vi "Inst_K2002.vi"(8 "error in":errorcluster, 10 "All Message Queues in":T1, 11 "Prueba31 in":refnum<class "Prueba06.lvclass">) -> (0 "error out":errorcluster)   [LabVIEW 2019, in "Prueba06.lvclass"]
uses:
  Prueba06.lvclass
  QMH/Message Queue/All Message Queues.ctl
  QMH/Message Queue/Message Cluster.ctl
  Prueba06.lvclass/Prueba06.ctl
  <vilib>/Utility/error.llb/Error Cluster From Error Code.vi
  QMH/Message Queue/Enqueue Message (Single).vi
  <vilib>/ErrorRing/Error Ring.xnode
  QMH/Message Queue/Message Queue.lvlib
  Instrumento/Keithley2002/Keithley2002.lvclass
panel:
  out "All States":string[](array[string])
  out "Actual State":string
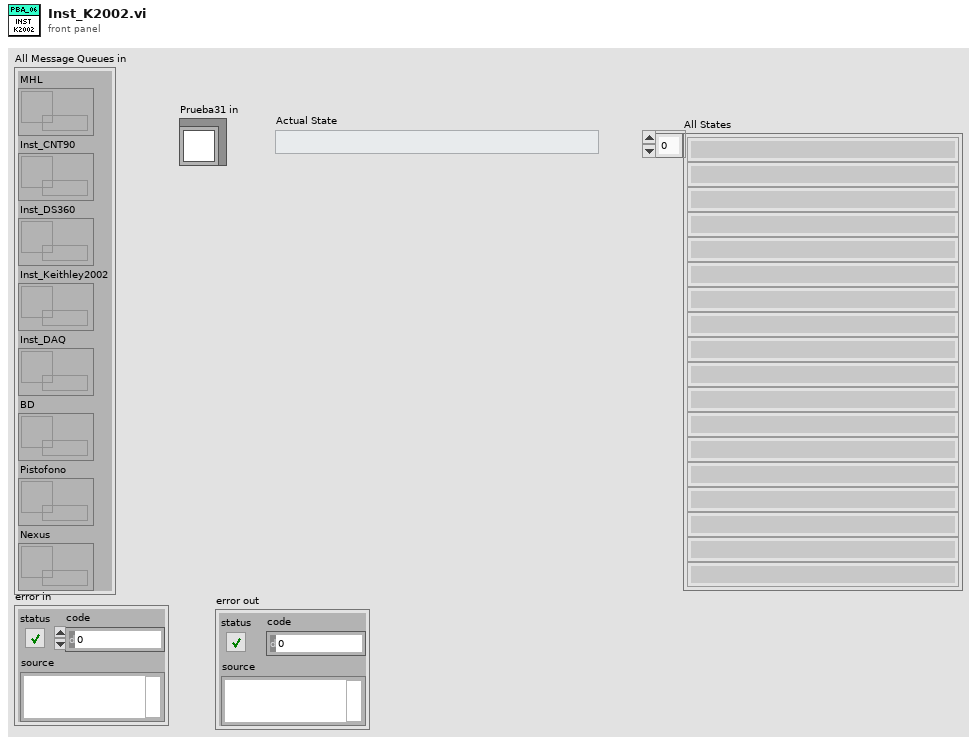
[diagram p1: front panel]
types:
  T1 = typedef "Message Queue.lvlib/All Message Queues.ctl" = cluster{"MHL":refnum<queue>, "Inst_CNT90":refnum<queue>, "Inst_DS360":refnum<queue>, "Inst_Keithley2002":refnum<queue>, "Inst_DAQ":refnum<queue>, "BD":refnum<queue>, "Pistofono":refnum<queue>, "Nexus":refnum<queue>}
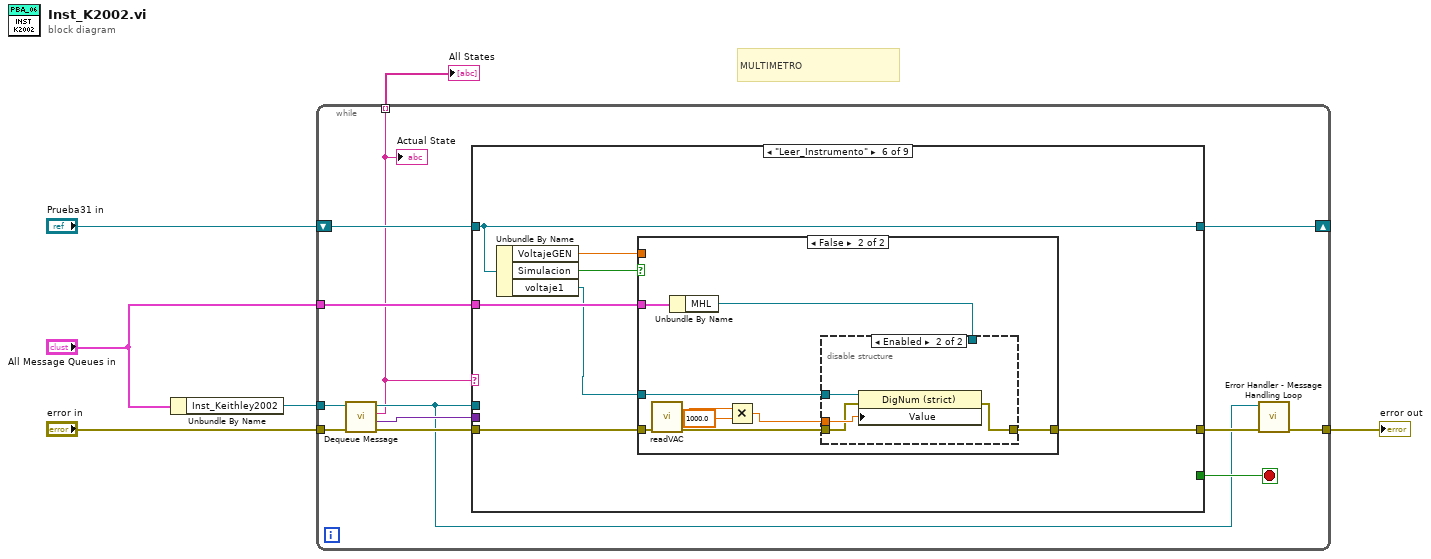
[diagram p0: block diagram]
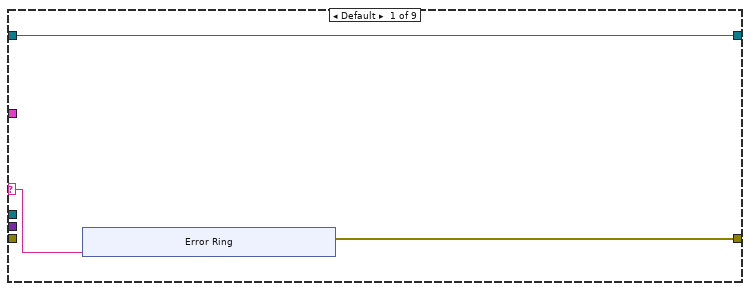
[diagram p2: hidden frame]
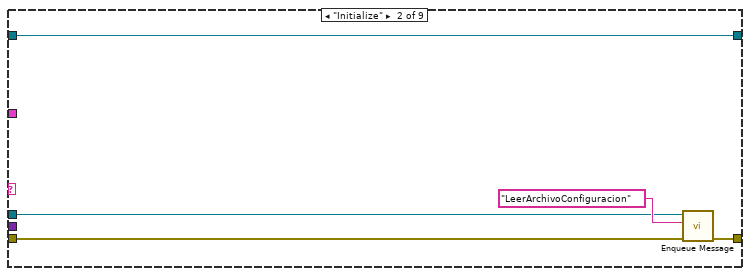
[diagram p3: hidden frame]
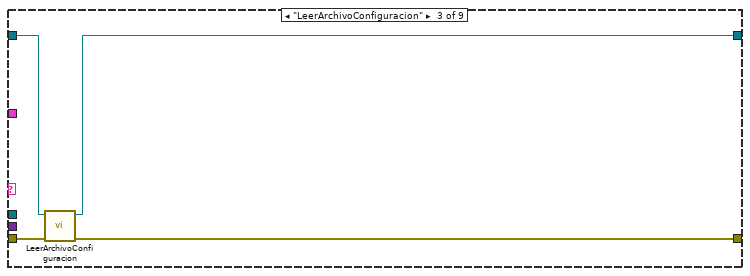
[diagram p4: hidden frame]
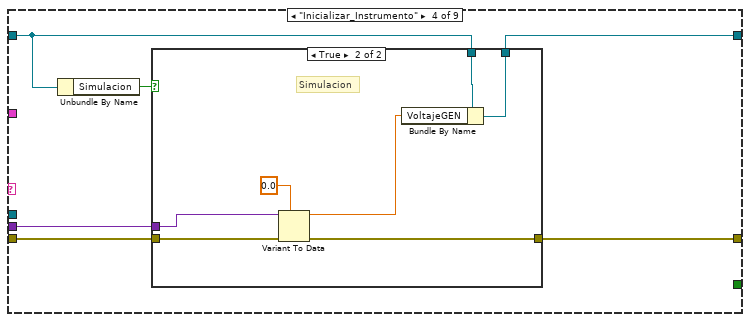
[diagram p5: hidden frame]
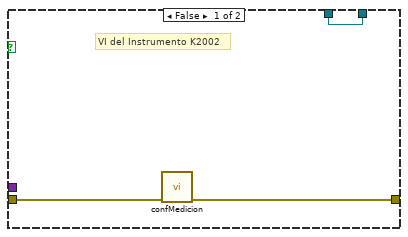
[diagram p6: hidden frame]
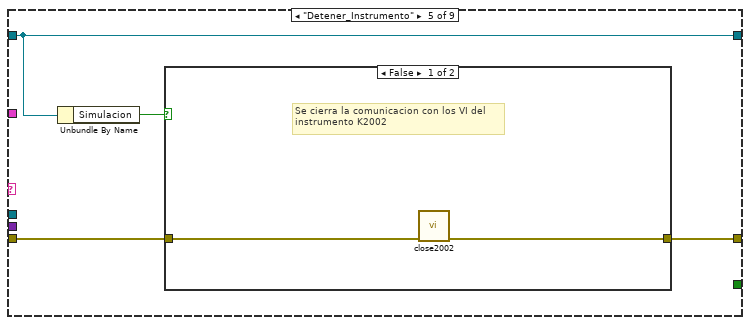
[diagram p7: hidden frame]
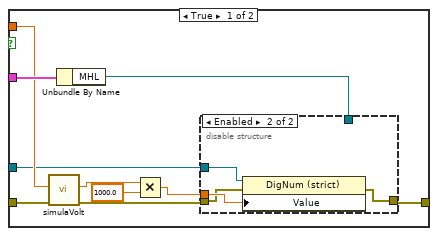
[diagram p9: hidden frame]
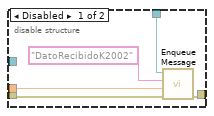
[diagram p10: hidden frame]
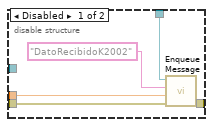
[diagram p11: hidden frame]
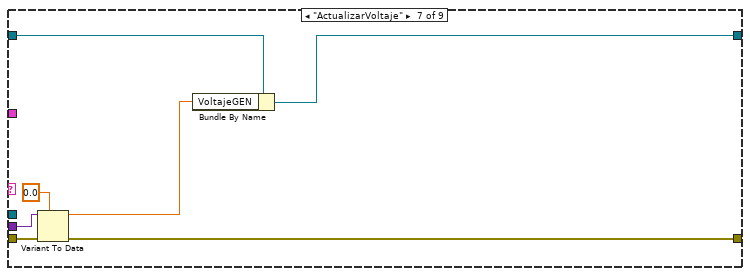
[diagram p12: hidden frame]
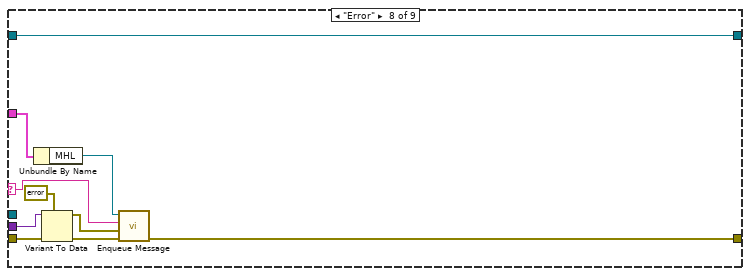
[diagram p13: hidden frame]
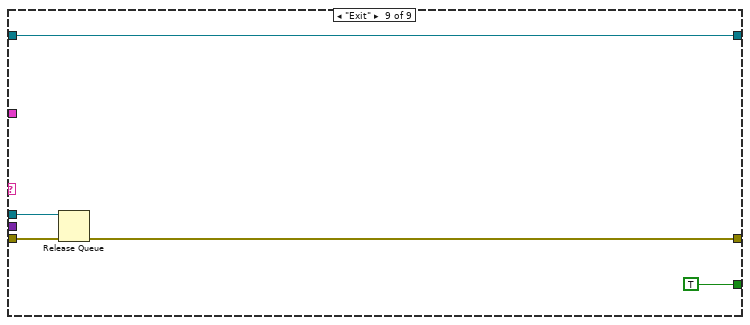
[diagram p14: hidden frame]
diagram:
  # "MULTIMETRO"
  n1 = Unbundle By Name("All Message Queues in") -> ("Inst_Keithley2002"=w4:refnum<queue>)
  n2 = while {
    tunnel: "error in" -> [w18]
    tunnel: w4 -> [w17]
    tunnel: "All Message Queues in" -> [w16]
    tunnel: [w9] -> w2
    shift-right: [w12] -> _
    shift-left: "Prueba31 in" -> [w15]
    tunnel: [w7] -> w1 mode=indexing
    stop <- w11 stop-if-true
    n3 = call "Dequeue Message.vi"("error in (no error)"=w18, "Message Queue"=w17) -> ("error out"=w13:errorcluster, "Message Data"=w14:variant, "Message"=w7:string, "dup Message Queue"=w8:refnum<queue>)  [unwired: 6 in]
    "Actual State" <- w7
    n4 = case shown="\"Leer_Instrumento\"" w7 {
      selector: w7 -> [w21 _ _ _ _ _ _ w114 _]
      tunnel: w16 -> [_ _ _ _ _ w65 _ w113 _]
      tunnel: w15 -> [w19 w33 w34 w40 w56 w67 w106 w121 w123]
      tunnel: w8 -> [_ w29 _ _ _ _ _ _ w125]
      tunnel: w14 -> [_ _ _ w38 _ _ w108 w118 _]
      tunnel: w13 -> [_ w31 w36 w41 w54 w64 w110 w119 w126]
      tunnel: [w20 w30 w37 w43 w57 w63 w111 w116 w122] -> w10
      tunnel: [w19 w33 w35 w39 w56 w67 w107 w121 w123] -> w12
      tunnel: [_ _ _ _ _ _ _ _ TRUE] -> w11
      frame Default {
        n5 = xnode "Error Ring"("parameter 0"=w21) -> ("error out"=w20:errorcluster)
      }
      frame "Initialize" {
        n6 = call-poly "Enqueue Message.vi"("error in (no error)"=w31, "Message"="LeerArchivoConfiguracion", "Message Queue"=w29) -> ("error out"=w30:errorcluster)  [unwired: 7 in, 1 out]
      }
      frame "LeerArchivoConfiguracion" {
        n7 = call "LeerArchivoConfiguracion.vi"("error in"=w36, "Prueba06 in"=w34) -> ("error out"=w37:errorcluster, "Prueba06 out"=w35:refnum<class "Prueba06.lvclass">)  [unwired: 8 in]
      }
      frame "Inicializar_Instrumento" {
        n8 = Unbundle By Name(w40) -> ("Simulacion"=w42:bool)
        n9 = case shown="True" w42 {
          tunnel: [w46 w50] -> w43
          tunnel: w41 -> [w45 w53]
          tunnel: w40 -> [w44 w52]
          tunnel: [w44 w51] -> w39
          tunnel: w38 -> [_ w49]
          frame False {
            # "VI del Instrumento K2002"
            n10 = call "confMedicion.vi"("error in (no error)"=w45) -> ("error out"=w46:errorcluster)  [unwired: 9 in, 1 out]
          }
          frame True {
            # "Simulacion"
            n11 = Variant To Data(error in=w53, type=0.0, Variant=w49) -> (data=w47:dbl, error out=w50:errorcluster)
            n12 = Bundle By Name(cluster=w52, "VoltajeGEN"=w47) -> (w51:refnum<class "Prueba06.lvclass">)
          }
        }
      }
      frame "Detener_Instrumento" {
        n13 = Unbundle By Name(w56) -> ("Simulacion"=w55:bool)
        n14 = case shown="False" w55 {
          tunnel: [w59 w60] -> w57
          tunnel: w54 -> [w58 w60]
          frame False {
            # "Se cierra la comunicacion con los VI del\ninstrumento K2002"
            n15 = call "close2002.vi"("error in (no error)"=w58) -> ("error out"=w59:errorcluster)  [unwired: 9 in, 1 out]
          }
          frame True {
            # "Simulacion"
          }
        }
      }
      frame "Leer_Instrumento" {
        n16 = Unbundle By Name(w67) -> ("VoltajeGEN"=w62:dbl, "Simulacion"=w66:bool, "voltaje1"=w61:refnum<vi>)
        n17 = case shown="False" w66 {
          tunnel: w65 -> [w77 w95]
          tunnel: [w74 w94] -> w63
          tunnel: w64 -> [w76 w92]
          tunnel: w62 -> [w72 _]
          tunnel: w61 -> [w71 w90]
          frame True {
            n18 = call "simulaVolt.vi"("error in (no error)"=w76, "volt in"=w72) -> ("error out"=w75:errorcluster, "volt out"=w70:dbl)  [unwired: 7 in, 1 out]
            n19 = Unbundle By Name(w77) -> ("MHL"=w73:refnum<queue>)
            n20 = Multiply(x=w70, y=1000.0) -> (x*y=w68:dbl)
            n21 = disable-structure shown="Enabled" {
              disable-tunnel: w75 -> [w82 w85]
              disable-tunnel: [w81 w84] -> w74
              disable-tunnel: w73 -> [w80 _]
              disable-tunnel: w68 -> [w78 w86]
              disable-tunnel: w71 -> [_ w83]
              frame Disabled {
                n22 = call-poly "Enqueue Message.vi"("error in (no error)"=w82, "Message Data"=w78, "Message"="DatoRecibidoK2002", "Message Queue"=w80) -> ("error out"=w81:errorcluster)  [unwired: 6 in, 1 out]
              }
              frame Enabled {
                n23 = property class="DigNum (strict)"(reference=w83, error in=w85, "Value"=w86) -> (error out=w84:errorcluster)  [unwired: 1 out]
              }
            }
          }
          frame False {
            n24 = call "readVAC.vi"("error in (no error)"=w92) -> ("error out"=w91:errorcluster, "medicion"=w89:dbl)  [unwired: 7 in, 2 out]
            n25 = Unbundle By Name(w95) -> ("MHL"=w93:refnum<queue>)
            n26 = Multiply(x=w89, y=1000.0) -> (x*y=w87:dbl)
            n27 = disable-structure shown="Enabled" {
              disable-tunnel: [w100 w101] -> w94
              disable-tunnel: w93 -> [w99 _]
              disable-tunnel: w91 -> [w97 w102]
              disable-tunnel: w87 -> [w96 w103]
              disable-tunnel: w90 -> [_ w104]
              frame Disabled {
                n28 = call-poly "Enqueue Message.vi"("error in (no error)"=w97, "Message Data"=w96, "Message"="DatoRecibidoK2002", "Message Queue"=w99) -> ("error out"=w100:errorcluster)  [unwired: 6 in, 1 out]
              }
              frame Enabled {
                n29 = property class="DigNum (strict)"(reference=w104, error in=w102, "Value"=w103) -> (error out=w101:errorcluster)  [unwired: 1 out]
              }
            }
          }
        }
      }
      frame "ActualizarVoltaje" {
        n30 = Variant To Data(error in=w110, type=0.0, Variant=w108) -> (data=w105:dbl, error out=w111:errorcluster)
        n31 = Bundle By Name(cluster=w106, "VoltajeGEN"=w105) -> (w107:refnum<class "Prueba06.lvclass">)
      }
      frame "Error" {
        n32 = Unbundle By Name(w113) -> ("MHL"=w112:refnum<queue>)
        n33 = Variant To Data(error in=w119, type=errorcluster {"status"=FALSE, "code"=0, "source"=""} ("error constant"), Variant=w118) -> (data=w115:errorcluster, error out=w117:errorcluster)
        n34 = call-poly "Enqueue Message.vi"("error in (no error)"=w117, "Message Data"=w115, "Message"=w114, "Message Queue"=w112) -> ("error out"=w116:errorcluster)  [unwired: 6 in, 1 out]
      }
      frame "Exit" {
        n35 = Release Queue(queue=w125, error in (no error)=w126) -> (error out=w122:errorcluster)  [unwired: 1 in, 2 out]
      }
    }
    n36 = call "Error Handler - Message Handling Loop.vi"("error in (no error)"=w10, "Message Queue"=w8) -> ("dup error in"=w9:errorcluster)  [unwired: 8 in, 1 out]
  }
  "error out" <- w2
  "All States" <- w1
